vi "fgv_total_roi_time.vi"(6 "Cycle Time with MC":dbl, 7 "Op":T1, 8 "error in (no error)":errorcluster, 9 "Cycle Time":dbl, 10 "Cycle Rate":dbl, 11 "Total cycle time":dbl) -> (0 "error out":errorcluster, 1 "Cycle Time":dbl, 2 "Cycle Rate":dbl, 3 "Total cycle time":dbl, 4 "Cycle Time with MC":dbl)   [LabVIEW 2020]
uses:
  Typedefs/FGV ROI Time Ops.ctl
panel:
  # "NOTE : THIS FGV IS ONLY BEING USED \nTO DETECT CHANGE IN ROIS THAT\nCAUSE CHANGE IN CYCLE TIME.\nTHE VALUE HELD IS ONLY FOR DEBUGGING.\nIT IS NOT USED FOR CYCLE RATE CALCULATION!!!"
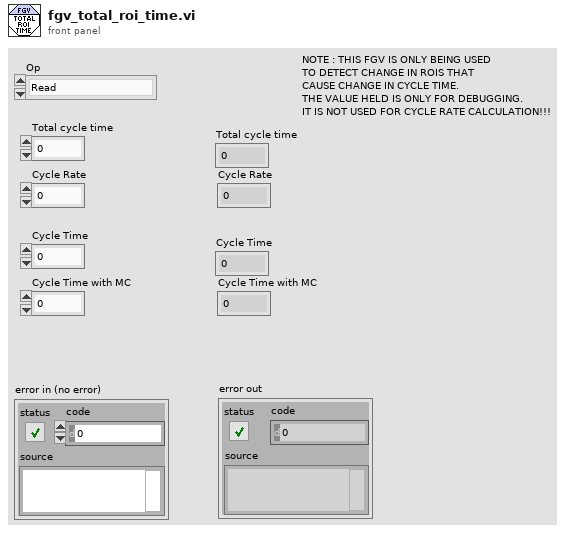
[diagram p1: front panel]
types:
  T1 = typedef "FGV ROI Time Ops.ctl" = enum16{"Read", "Write Cycle Time", "Write Cycle Rate"}
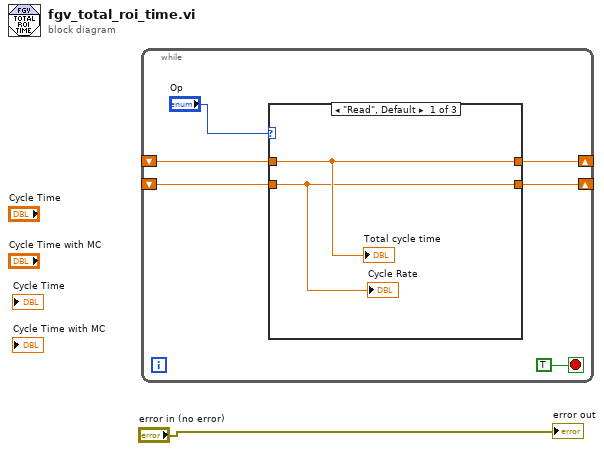
[diagram p0: block diagram]
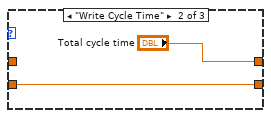
[diagram p2: hidden frame]
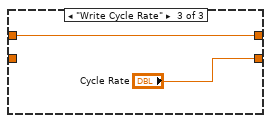
[diagram p3: hidden frame]
diagram:
  n1 = while {
    shift-right: [w7] -> _
    shift-left: _ -> [w6]
    shift-right: [w5] -> _
    shift-left: _ -> [w4]
    stop <- TRUE stop-if-true
    n2 = case shown="\"Read\", Default" "Op" {
      tunnel: [w9 "Total cycle time" w13] -> w7
      tunnel: w6 -> [w9 _ w13]
      tunnel: [w8 w10 "Cycle Rate"] -> w5
      tunnel: w4 -> [w8 w10 _]
      frame "Read", Default {
        "Total cycle time" <- w9
        "Cycle Rate" <- w8
      }
      frame "Write Cycle Time" {
      }
      frame "Write Cycle Rate" {
      }
    }
  }
  "error out" <- "error in (no error)"
